vi "Generate Sqare Wave.vi"(8 "error in (no error)":errorcluster, 11 "Sq Wave Properties":T1 {"Duty Cycle(%)" min=0 max=100}) -> (0 "error out":errorcluster, 3 "Waveform":waveform(dbl)(graph))   [LabVIEW 2017]
doc: "This VI gets the information from Square Wave Properties and converts them to an actual waveform that is readable by the DAQ.\n\nThis VI uses the default generate Square Wave VI from LabVIEW. The maths involved involved in the inputs are based from the properties of the DAQ Task that connects to the drive. I believe that the name of this DAQ Task is \"PrecorPulsedRPM\"."
uses:
  <vilib>/measure/NI_MABase.lvlib
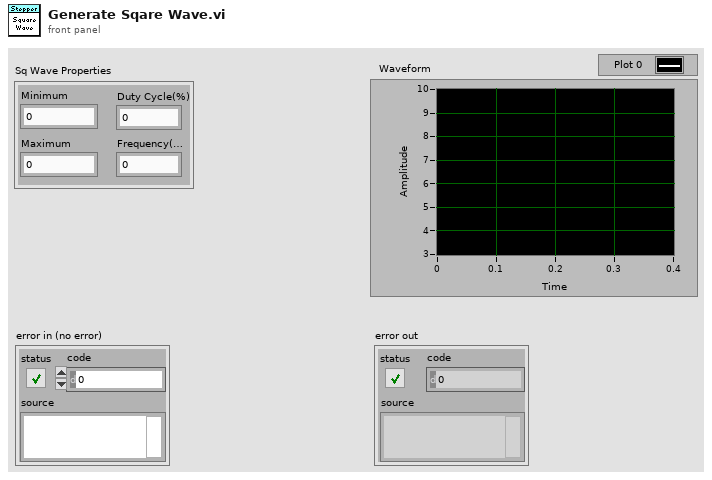
[diagram p1: front panel]
types:
  T1 = cluster{"Minimum":sgl, "Maximum":sgl, "Duty Cycle(%)":sgl, "Frequency(Hz))":sgl}
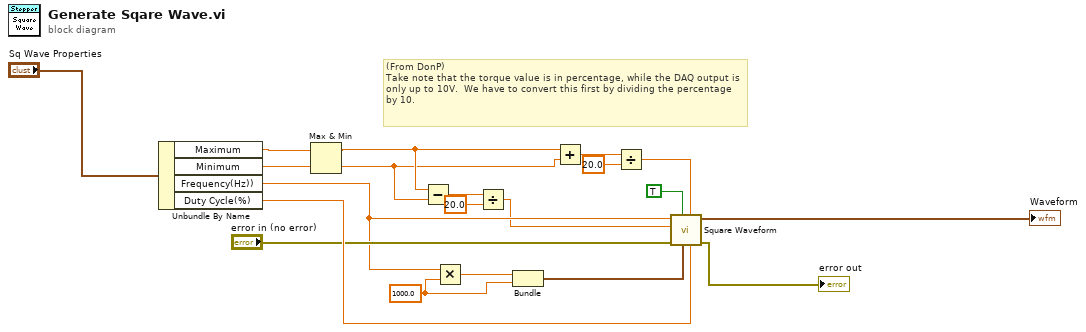
[diagram p0: block diagram]
diagram:
  w16 = 1000.0 ("y")
  # "(From DonP)\nTake note that the torque value is in percentage, while the DAQ output is only up to 10V.  We have to convert this first by dividing the percentage by 10."
  n1 = Unbundle By Name("Sq Wave Properties") -> ("Maximum"=w7:sgl, "Minimum"=w6:sgl, "Frequency(Hz))"=w11:sgl, "Duty Cycle(%)"=w17:sgl)
  n2 = Max & Min(x=w7, y=w6) -> (max(x,y)=w2:sgl, min(x,y)=w1:sgl)
  n3 = Subtract(x=w2, y=w1) -> (x-y=w10:sgl)
  n4 = Multiply(x=w11, y=w16) -> (x*y=w12:dbl)
  n5 = Divide(x=w10, y=sgl 20.0) -> (x/y=w8:sgl)
  n6 = Bundle(w12, "y"=w16) -> (w15:cluster{dbl, "y":dbl})  [unwired: 1 in]
  n7 = Add(x=w2, y=w1) -> (x+y=w5:sgl)
  n8 = Divide(x=w5, y=sgl 20.0) -> (x/y=w4:sgl)
  n9 = call <vilib>:"Square Waveform.vi"("duty cycle (%)"=w17, "offset"=w4, "sampling info"=w15, "reset signal"=TRUE, "error in (no error)"="error in (no error)", "amplitude"=w8, "frequency"=w11) -> ("error out"=→"error out":errorcluster, "signal out"=→"Waveform":waveform(dbl))  [unwired: 3 in]
